vi "WinHostToFlexRIO.vi"() -> ()   [LabVIEW 2013]
uses:
  <vilib>/userdefined/High Color/nirio_resource_hc.ctl
  <vilib>/FPGAPlugInAG/PXIe-7966R/niLvFpga_Open_PXIe-7966R.vi
  <vilib>/FPGAPlugInAG/PXIe-7966R/niLvFpga_Reset_PXIe-7966R.vi
  <vilib>/Utility/error.llb/Error Cluster From Error Code.vi
  <vilib>/rvi/errors/niLvFpgaAdjustHostInterfaceError.vi
  <vilib>/FPGAPlugInAG/PXIe-7966R/niLvFpga_Run_PXIe-7966R.vi
  <vilib>/rvi/interface/common/niFpgaWaitOnOcc.vi
  <vilib>/FPGAPlugInAG/PXIe-7966R/niLvFpga_Close_PXIe-7966R.vi
  <vilib>/rvi/interface/nirviOpenFPGA/nirviOpenFPGA.xnode
  FPGA Bitfiles/PXIe-7966R-FlexRIOnoModule_v1_1.lvbitx
  <vilib>/rvi/interface/nirviMethod/nirviMethod.xnode
  <vilib>/rvi/interface/nirviReadWriteControl/nirviReadWriteControl.xnode
  Control 1.ctl
  <vilib>/rvi/interface/nirviCloseFPGA/nirviCloseFPGA.xnode
  <vilib>/rvi/errors/niLvFpgaMergeErrorWithErrorCode.vi
  NiFpgaLv.dll
  <vilib>/FPGAPlugInAG/PXIe-7966R/niLvFpga_ConfigureFifo_PXIe-7966R.vi
  <vilib>/FPGAPlugInAG/PXIe-7966R/niLvFpga_StartFifo_PXIe-7966R.vi
panel:
  out "auxAI5":i32
  out "auxAI4":i32
  out "auxAI3":i32
  out "auxAI2":i32
  out "auxAI1":i32
  out "auxAI0":i32
  in  "auxAO5":i32
  in  "auxAO4":i32
  in  "auxAO3":i32
  in  "auxAO2":i32
  in  "auxAO1":i32
  in  "auxAO0":i32
  in  "FlexRIO device":T1
  in  "stop":bool
  out "auxDI5":bool
  out "auxDI4":bool
  out "auxDI3":bool
  out "auxDI2":bool
  out "auxDI1":bool
  out "auxDI0":bool
  in  "auxDO5":bool
  in  "auxDO4":bool
  in  "auxDO3":bool
  in  "auxDO2":bool
  in  "auxDO1":bool
  in  "auxDO0":bool
  out "error out":errorcluster
  out "DMATtoHOSTBlockNWords":u16[](array[numeric])
  out "DMATtoHOSTSampleSize":u8[](array[numeric])
  out "DMATtoHOSTNCh":u16[](array[numeric])
  out "DMATtoHOSTFrameType":u8[](array[numeric])
  out "DevProfile":u8
  out "DevTemp":i16
  out "DevQualityStatus":u8
  out "Fref":u32
  out "RIOAdapterCorrect":bool
  out "Expected IO Module ID":u32
  out "InsertedIOModule ID":u32
  out "FPGAVIversion":u8[](array[numeric])
  out "Platform":enum8{"FlexRIO", "cRIO", "RSeries"}(ring)
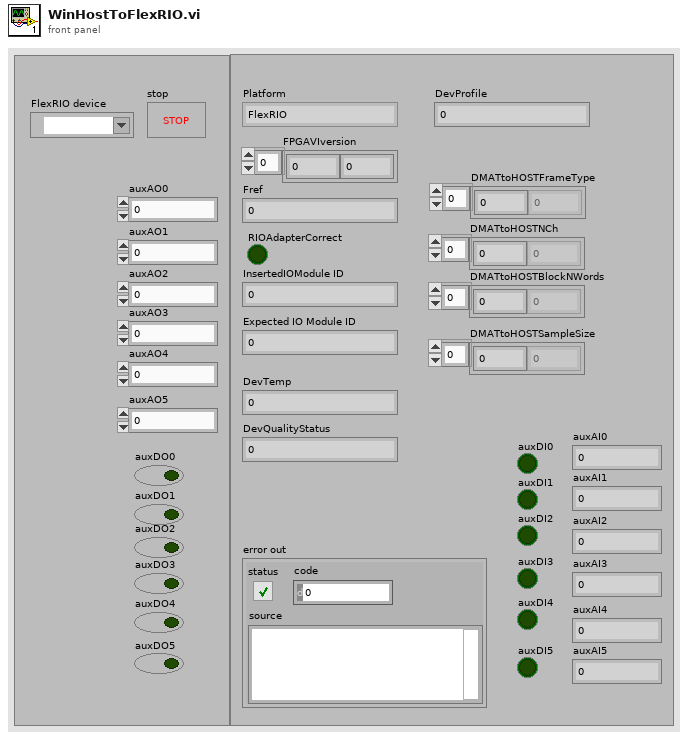
[diagram p1: front panel]
types:
  T1 = typedef "nirio_resource_hc.ctl" = tag
  T2 = enum16{"DAQ-CPU", "IMAQ-CPU", "DAQ-GPU", "IMAQ-GPU"}
  T3 = typedef "Control 1.ctl" = u16
  T4 = cluster{"Timeout":u8, "Timeout":T3, "Timeout":u8, "Timeout":u16}
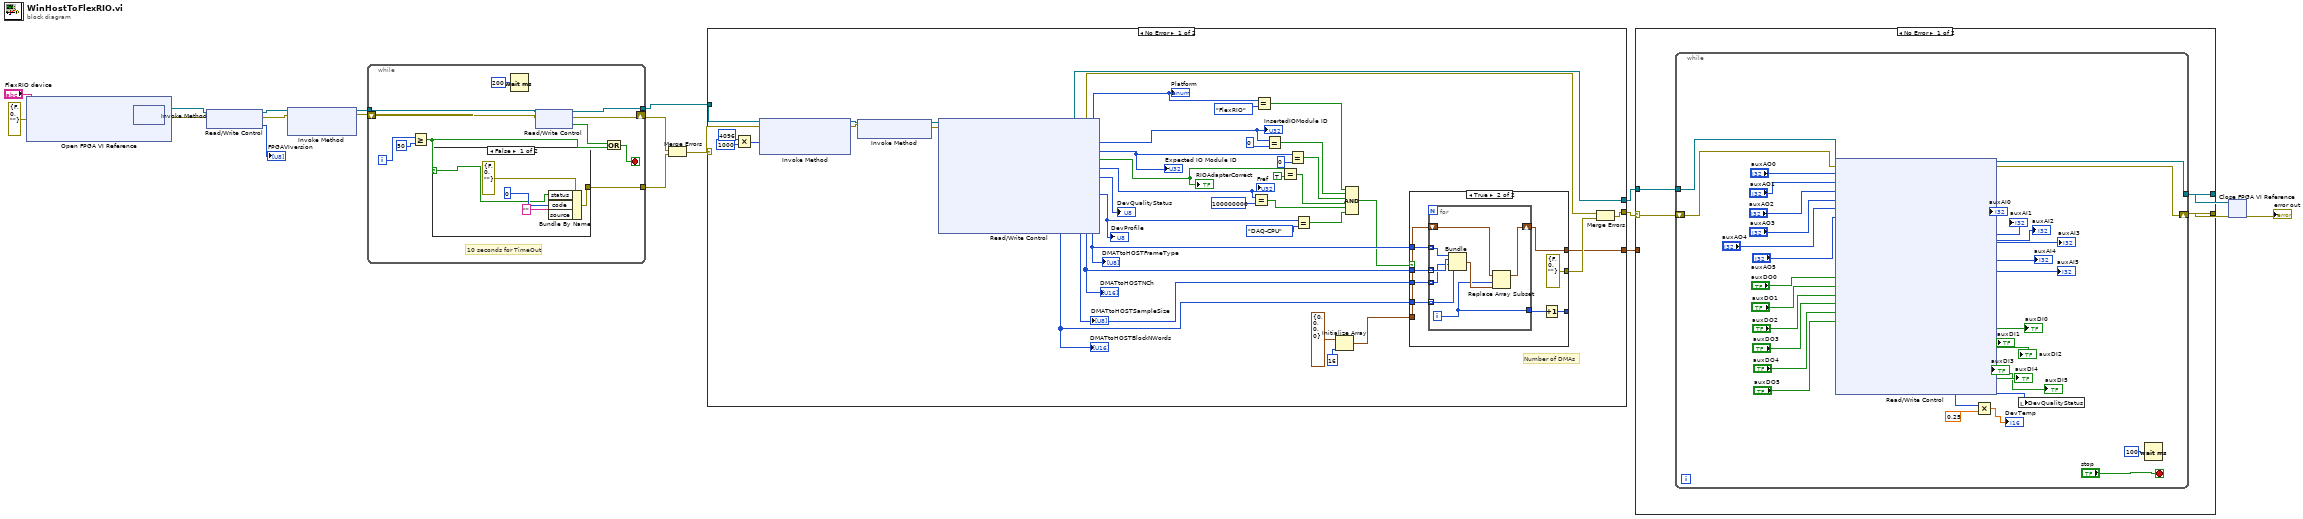
[diagram p0: block diagram]
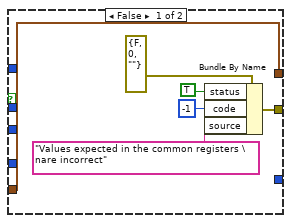
[diagram p3: hidden frame]
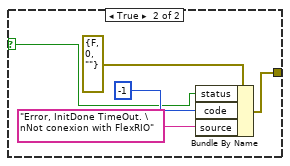
[diagram p5: hidden frame]
diagram:
  n1 = xnode "Open FPGA VI Reference"("error in"=errorcluster {"status"=FALSE, "code"=0, "source"=""}, "resource name"="FlexRIO device") -> ("FPGA VI Reference Out"=w20:refnum<k20>, "error out"=w21:errorcluster)
  n2 = xnode "Invoke Method"("FPGA VI Reference In"=w20, "error in"=w21) -> ("FPGA VI Reference Out"=w5:refnum<k20>, "error out"=w4:errorcluster)
  n3 = xnode "Read/Write Control"("FPGA VI Reference In"=w5, "error in"=w4) -> ("FPGA VI Reference Out"=w3:refnum<k20>, "error out"=w2:errorcluster, "FPGAVIversion"=→"FPGAVIversion":u8[])
  n4 = xnode "Invoke Method"("FPGA VI Reference In"=w3, "error in"=w2) -> ("FPGA VI Reference Out"=w18:refnum<k20>, "error out"=w17:errorcluster)  [unwired: 1 in]
  n5 = while {
    tunnel: w18 -> [w32]
    tunnel: [w29] -> w16
    shift-right: [w30] -> w14
    shift-left: w17 -> [w31]
    tunnel: [w22] -> w15
    i -> [w27]
    stop <- w24 stop-if-true
    # "10 seconds for TimeOut"
    n6 = Greater Or Equal?(x=w27, y=50) -> (x >= y?=w23:bool)
    n7 = case shown="False" w23 {
      selector: w23 -> [w34 w39]
      tunnel: [w33 w38] -> w22
      frame False {
        n8 = Bundle By Name(cluster=errorcluster {"status"=FALSE, "code"=0, "source"=""} ("error constant"), "status"=w34, "code"=0, "source"="") -> (w33:errorcluster)
      }
      frame True {
        n9 = Bundle By Name(cluster=errorcluster {"status"=FALSE, "code"=0, "source"=""} ("error constant"), "status"=w39, "code"=-1, "source"="Error, InitDone TimeOut. \nNot conexion with FlexRIO") -> (w38:errorcluster)
      }
    }
    n10 = Wait (ms)(milliseconds to wait=u32 200) -> ()  [unwired: 1 out]
    n11 = xnode "Read/Write Control"("FPGA VI Reference In"=w32, "error in"=w31) -> ("FPGA VI Reference Out"=w29:refnum<k20>, "error out"=w30:errorcluster, "InitDone"=w25:bool)
    n12 = Or(x=w25, y=w23) -> (x .or. y?=w24:bool)
  }
  n13 = Merge Errors(w14, w15) -> (w13:errorcluster)
  n14 = case shown="No Error" w13 {
    selector: w13 -> [w77 w108]
    tunnel: w16 -> [w78 w107]
    tunnel: [w73 w107] -> w10
    tunnel: [w45 w108] -> w11
    tunnel: [w43 _] -> w7
    frame No Error {
      # "Number of DMAs"
      n15 = Multiply(x=u32 4096 ("Requested Depth"), y=u32 1000) -> (x*y=w79:u32)
      n16 = xnode "Invoke Method"("FPGA VI Reference In"=w78, "error in"=w77, "Requested Depth"=w79) -> ("FPGA VI Reference Out"=w83:refnum<k20>, "error out"=w82:errorcluster)  [unwired: 1 out]
      n17 = xnode "Invoke Method"("FPGA VI Reference In"=w83, "error in"=w82) -> ("FPGA VI Reference Out"=w75:refnum<k20>, "error out"=w76:errorcluster)
      n18 = xnode "Read/Write Control"("FPGA VI Reference In"=w75, "error in"=w76) -> ("FPGA VI Reference Out"=w73:refnum<k20>, "error out"=w46:errorcluster, "Platform"=w72:enum8{"FlexRIO", "cRIO", "RSeries"}, "InsertedIOModule ID"=w66:u32, "Expected IO Module ID"=w64:u32, "RIOAdapterCorrect"=w68:bool, "Fref"=w70:u32, "DevQualityStatus"=→"DevQualityStatus":u8, "DevProfile"=w62:u8, "DMATtoHOSTFrameType"=w57:u8[], "DMATtoHOSTNCh"=w60:T3[], "DMATtoHOSTSampleSize"=w59:u8[], "DMATtoHOSTBlockNWords"=w58:u16[])  [unwired: 1 out]
      "Platform" <- w72
      "InsertedIOModule ID" <- w66
      "Expected IO Module ID" <- w64
      "RIOAdapterCorrect" <- w68
      "Fref" <- w70
      "DevProfile" <- w62
      "DMATtoHOSTFrameType" <- w57
      "DMATtoHOSTNCh" <- w60
      "DMATtoHOSTSampleSize" <- w59
      "DMATtoHOSTBlockNWords" <- w58
      n19 = Equal?(x=w70, y=u32 100000000) -> (x = y?=w51:bool)
      n20 = Equal?(x=w72, y=enum16{"FlexRIO", "cRIO", "R-Series"}."FlexRIO") -> (x = y?=w55:bool)
      n21 = Equal?(x=w66, y=u32 0) -> (x = y?=w54:bool)
      n22 = Equal?(x=w68, y=TRUE) -> (x = y?=w52:bool)
      n23 = Equal?(x=w64, y=u32 0) -> (x = y?=w53:bool)
      n24 = Equal?(x=w62, y=T2."DAQ-CPU") -> (x = y?=w50:bool)
      n25 = Initialize Array(cluster{u8, u16, u8, u16} {0, 0, 0, 0}, 16 ("dimension size")) -> (w47:cluster{u8, u16, u8, u16}[])
      n26 = Compound Arithmetic op=AND(w55, w54, w53, w52, w51, w50) -> (w56:bool)
      n27 = case shown="True" w56 {
        tunnel: w60 -> [_ w98]
        tunnel: w59 -> [_ w97]
        tunnel: w58 -> [_ w96]
        tunnel: w57 -> [_ w95]
        tunnel: w47 -> [w84 w94]
        tunnel: [w84 w93] -> w43
        tunnel: [w85 errorcluster {"status"=FALSE, "code"=0, "source"=""} ("error constant")] -> w44
        tunnel: [_ w90] -> _
        frame False {
          n28 = Bundle By Name(cluster=errorcluster {"status"=FALSE, "code"=0, "source"=""} ("error constant"), "status"=TRUE, "code"=-1, "source"="Values expected in the common registers \nare incorrect") -> (w85:errorcluster)
        }
        frame True {
          n29 = for {
            tunnel: w98 -> [w104] mode=indexing
            tunnel: w97 -> [w103] mode=indexing
            tunnel: w96 -> [w102] mode=indexing
            tunnel: w95 -> [w105] mode=indexing
            shift-right: [w100] -> w93
            shift-left: w94 -> [w106]
            tunnel: [w99] -> w91
            i -> [w99]
            n30 = Bundle("Timeout"=w105, "Timeout"=w104, "Timeout"=w103, "Timeout"=w102) -> (w101:T4)  [unwired: 1 in]
            n31 = Replace Array Subset(array=w106, new element=w101, index=w99) -> (w100:cluster{u8, u16, u8, u16}[])
          }
          n32 = Increment(x=w91) -> (x+1=w90:i32)
        }
      }
      n33 = Merge Errors(w46, w44) -> (w45:errorcluster)
    }
    frame Error {
    }
  }
  n34 = case shown="No Error" w11 {
    selector: w11 -> [w109 w148]
    tunnel: w10 -> [w110 w147]
    tunnel: [w112 w147] -> w9
    tunnel: [w111 w148] -> w8
    tunnel: w7 -> [_ _]
    frame No Error {
      n35 = while {
        shift-right: [w131] -> w111
        shift-left: w109 -> [w145]
        tunnel: w110 -> [w146]
        tunnel: [w144] -> w112
        stop <- "stop" stop-if-true
        n36 = xnode "Read/Write Control"("FPGA VI Reference In"=w146, "error in"=w145, "auxAO0"="auxAO0", "auxAO1"="auxAO1", "auxAO2"="auxAO2", "auxAO3"="auxAO3", "auxAO4"="auxAO4", "auxAO5"="auxAO5", "auxDO0"="auxDO0", "auxDO1"="auxDO1", "auxDO2"="auxDO2", "auxDO3"="auxDO3", "auxDO4"="auxDO4", "auxDO5"="auxDO5") -> ("FPGA VI Reference Out"=w144:refnum<k20>, "error out"=w131:errorcluster, "auxAI0"=→"auxAI0":i32, "auxAI1"=→"auxAI1":i32, "auxAI2"=→"auxAI2":i32, "auxAI3"=→"auxAI3":i32, "auxAI4"=→"auxAI4":i32, "auxAI5"=→"auxAI5":i32, "auxDI0"=→"auxDI0":bool, "auxDI1"=→"auxDI1":bool, "auxDI2"=→"auxDI2":bool, "auxDI3"=→"auxDI3":bool, "auxDI4"=→"auxDI4":bool, "auxDI5"=→"auxDI5":bool, "DevQualityStatus"=w129:u8, "DevTemp"=w116:i16)
        n37 = Multiply(x=w116, y=0.25) -> (x*y=→"DevTemp":dbl)
        n38 = local write "DevQualityStatus"(w129) -> ()
        n39 = Wait (ms)(milliseconds to wait=u32 100) -> ()  [unwired: 1 out]
      }
    }
    frame Error {
    }
  }
  n40 = xnode "Close FPGA VI Reference"("FPGA VI Reference In"=w9, "error in"=w8) -> ("error out"=→"error out":errorcluster)
